vi "CLOSE.vi"(8 "error in (no error)":errorcluster, 11 "SIMULADO in":refnum<class "SIMULADO.lvclass">) -> (0 "error out":errorcluster, 3 "SIMULADO out":refnum<class "SIMULADO.lvclass">)   [LabVIEW 2019, in "SIMULADO.lvclass"]
uses:
  SIMULADO.lvclass
  SERIAL DEVICE/SERIAL DEVICE.lvclass
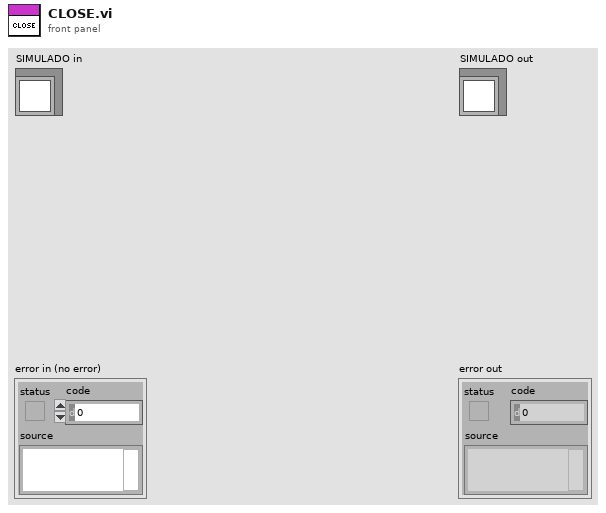
[diagram p1: front panel]
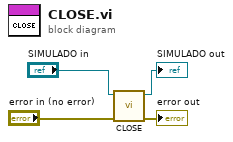
[diagram p0: block diagram]
diagram:
  n1 = call-parent "CLOSE.vi"("error in (no error)"="error in (no error)", "SERIAL DEVICE in"="SIMULADO in") -> ("error out"=→"error out":errorcluster, "SERIAL DEVICE out"=→"SIMULADO out":refnum<class "SIMULADO.lvclass">)  [unwired: 8 in]
